vi "PicoScope2000Open.vi"(9 "error in (no error)":errorcluster) -> (1 "Unit Info":T1, 2 "handle":i16, 3 "error out":errorcluster)   [LabVIEW 2010]
doc: "This VI opens a PicoScope 3000a/b and returns a handle to the device."
uses:
  ps2000.dll
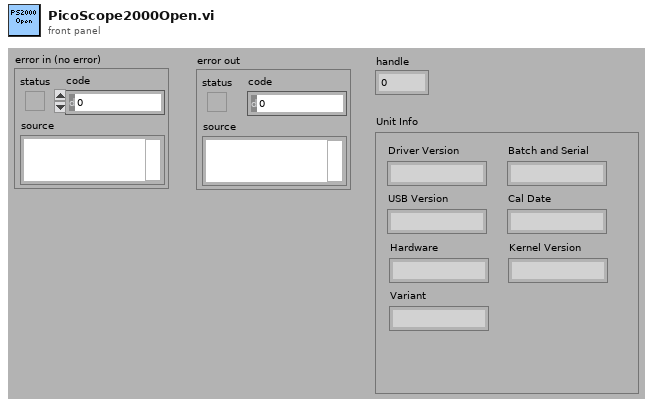
[diagram p1: front panel]
types:
  T1 = cluster{"Driver Version":string, "USB Version":string, "Hardware":string, "Variant":string, "Batch and Serial":string, "Cal Date":string, "Kernel Version":string}
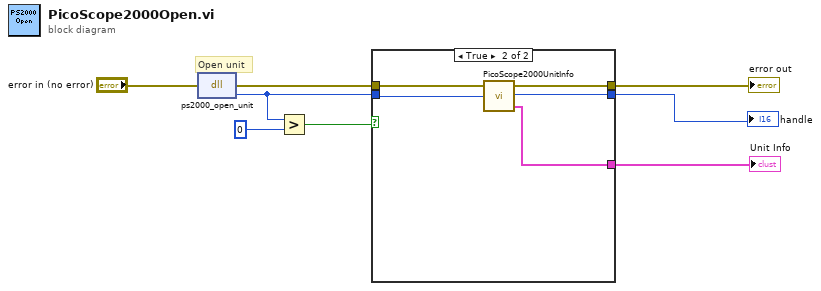
[diagram p0: block diagram]
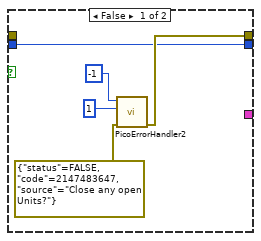
[diagram p2: hidden frame]
diagram:
  # "Open unit"
  n1 = dll-call lib="PS2000.dll" fn="ps2000_open_unit"(error in="error in (no error)") -> (error out=w7:errorcluster, "handle"=w2:i16)  [unwired: 2 in, 1 out]
  n2 = Greater?(x=w2, y=i16 0) -> (0:w3:bool)
  n3 = case shown="True" w3 {
    tunnel: w2 -> [w10 w14]
    tunnel: [w10 w15] -> w4
    tunnel: [w13 w16] -> w5
    tunnel: w7 -> [_ w17]
    tunnel: [_ w18] -> w6
    frame False {
      n4 = call "PicoErrorHandler2.vi"("error in (no error)"=errorcluster {"status"=FALSE, "code"=2147483647, "source"="Close any open Units?"}, "Default handle"=i16 1, "handle In"=i16 -1) -> ("error out"=w13:errorcluster)  [unwired: 8 in]
    }
    frame True {
      n5 = call "PicoScope2000UnitInfo.vi"("handle in"=w14, "error in (no error)"=w17) -> ("Unit Info"=w18:T1, "handle out"=w15:i16, "error out"=w16:errorcluster)  [unwired: 1 in]
    }
  }
  "handle" <- w4
  "error out" <- w5
  "Unit Info" <- w6
